vi "settings NM array.vi"(9 "Settings NM":dbl[](array[numeric]), 11 "Settings NM":T1 {"T8"."Medie" min=1 step=1; "T7"."Medie" min=1 step=1; "T6"."Medie" min=1 step=1; "T5"."Medie" min=1 step=1; "T4"."Medie" min=1 step=1; "T3"."Medie" min=1 step=1; "RM3"."Medie" min=1 step=1; "Tq3"."Medie" min=1 step=1; "Tq2"."Medie" min=1 step=1; "N3(T)"."Medie" min=1 step=1; "N2(T)"."Medie" min=1 step=1; "P10"."Medie" min=1 step=1; "P9"."Medie" min=1 step=1; "P8"."Medie" min=1 step=1; "P7"."Medie" min=1 step=1; "P6"."Medie" min=1 step=1; "P5"."Medie" min=1 step=1; "Q10"."Medie" min=1 step=1; "Q9"."Medie" min=1 step=1; "Q8"."Medie" min=1 step=1; "Q7"."Medie" min=1 step=1; "Q6"."Medie" min=1 step=1; "Q5"."Medie" min=1 step=1; "Pbar"."Medie" min=1 step=1; "Liv."."Medie" min=1 step=1; "RM2"."Medie" min=1 step=1; "RM1"."Medie" min=1 step=1; "T2"."Medie" min=1 step=1; "P4"."Medie" min=1 step=1; "Q4"."Medie" min=1 step=1; "RPM" items=["TESTO", "TORSIOMETRO", "OTTICA"]; "PRESSIONE\nMANDATA" items=["P1", "P2", "P3", "P4"]; "PRESSIONE\nASPIRAZIONE" items=["P1", "P2", "P3", "P4"]; "PORTATA\nSECONDARIA" items=["Q1", "Q2", "Q3", "Q4"]; "PORTATA\nPRINCIPALE" items=["LINEA ELETTROPOMPA", "LINEA SOMMERSA"]; "T1"."Medie" min=1 step=1; "Tq1"."Medie" min=1 step=1; "N1(T)"."Medie" min=1 step=1; "P3"."Medie" min=1 step=1; "P2"."Medie" min=1 step=1; "P1"."Medie" min=1 step=1; "Q3"."Medie" min=1 step=1; "Q2"."Medie" min=1 step=1; "Q1"."Medie" min=1 step=1}) -> (1 "Settings NM out":T1 {"T8"."Medie" min=1 step=1; "T7"."Medie" min=1 step=1; "T6"."Medie" min=1 step=1; "T5"."Medie" min=1 step=1; "T4"."Medie" min=1 step=1; "T3"."Medie" min=1 step=1; "RM3"."Medie" min=1 step=1; "Tq3"."Medie" min=1 step=1; "Tq2"."Medie" min=1 step=1; "N3(T)"."Medie" min=1 step=1; "N2(T)"."Medie" min=1 step=1; "P10"."Medie" min=1 step=1; "P9"."Medie" min=1 step=1; "P8"."Medie" min=1 step=1; "P7"."Medie" min=1 step=1; "P6"."Medie" min=1 step=1; "P5"."Medie" min=1 step=1; "Q10"."Medie" min=1 step=1; "Q9"."Medie" min=1 step=1; "Q8"."Medie" min=1 step=1; "Q7"."Medie" min=1 step=1; "Q6"."Medie" min=1 step=1; "Q5"."Medie" min=1 step=1; "Pbar"."Medie" min=1 step=1; "Liv."."Medie" min=1 step=1; "RM2"."Medie" min=1 step=1; "RM1"."Medie" min=1 step=1; "T2"."Medie" min=1 step=1; "P4"."Medie" min=1 step=1; "Q4"."Medie" min=1 step=1; "RPM" items=["TESTO", "TORSIOMETRO", "OTTICA"]; "PRESSIONE\nMANDATA" items=["P1", "P2", "P3", "P4"]; "PRESSIONE\nASPIRAZIONE" items=["P1", "P2", "P3", "P4"]; "PORTATA\nSECONDARIA" items=["Q1", "Q2", "Q3", "Q4"]; "PORTATA\nPRINCIPALE" items=["LINEA ELETTROPOMPA", "LINEA SOMMERSA"]; "T1"."Medie" min=1 step=1; "Tq1"."Medie" min=1 step=1; "N1(T)"."Medie" min=1 step=1; "P3"."Medie" min=1 step=1; "P2"."Medie" min=1 step=1; "P1"."Medie" min=1 step=1; "Q3"."Medie" min=1 step=1; "Q2"."Medie" min=1 step=1; "Q1"."Medie" min=1 step=1}, 3 "Settings NM out":dbl[](array[numeric]))   [LabVIEW 2019]
uses:
  TypeDef/cDAQ Settings NM.ctl
  TypeDef/SETUP INGRESSO.ctl
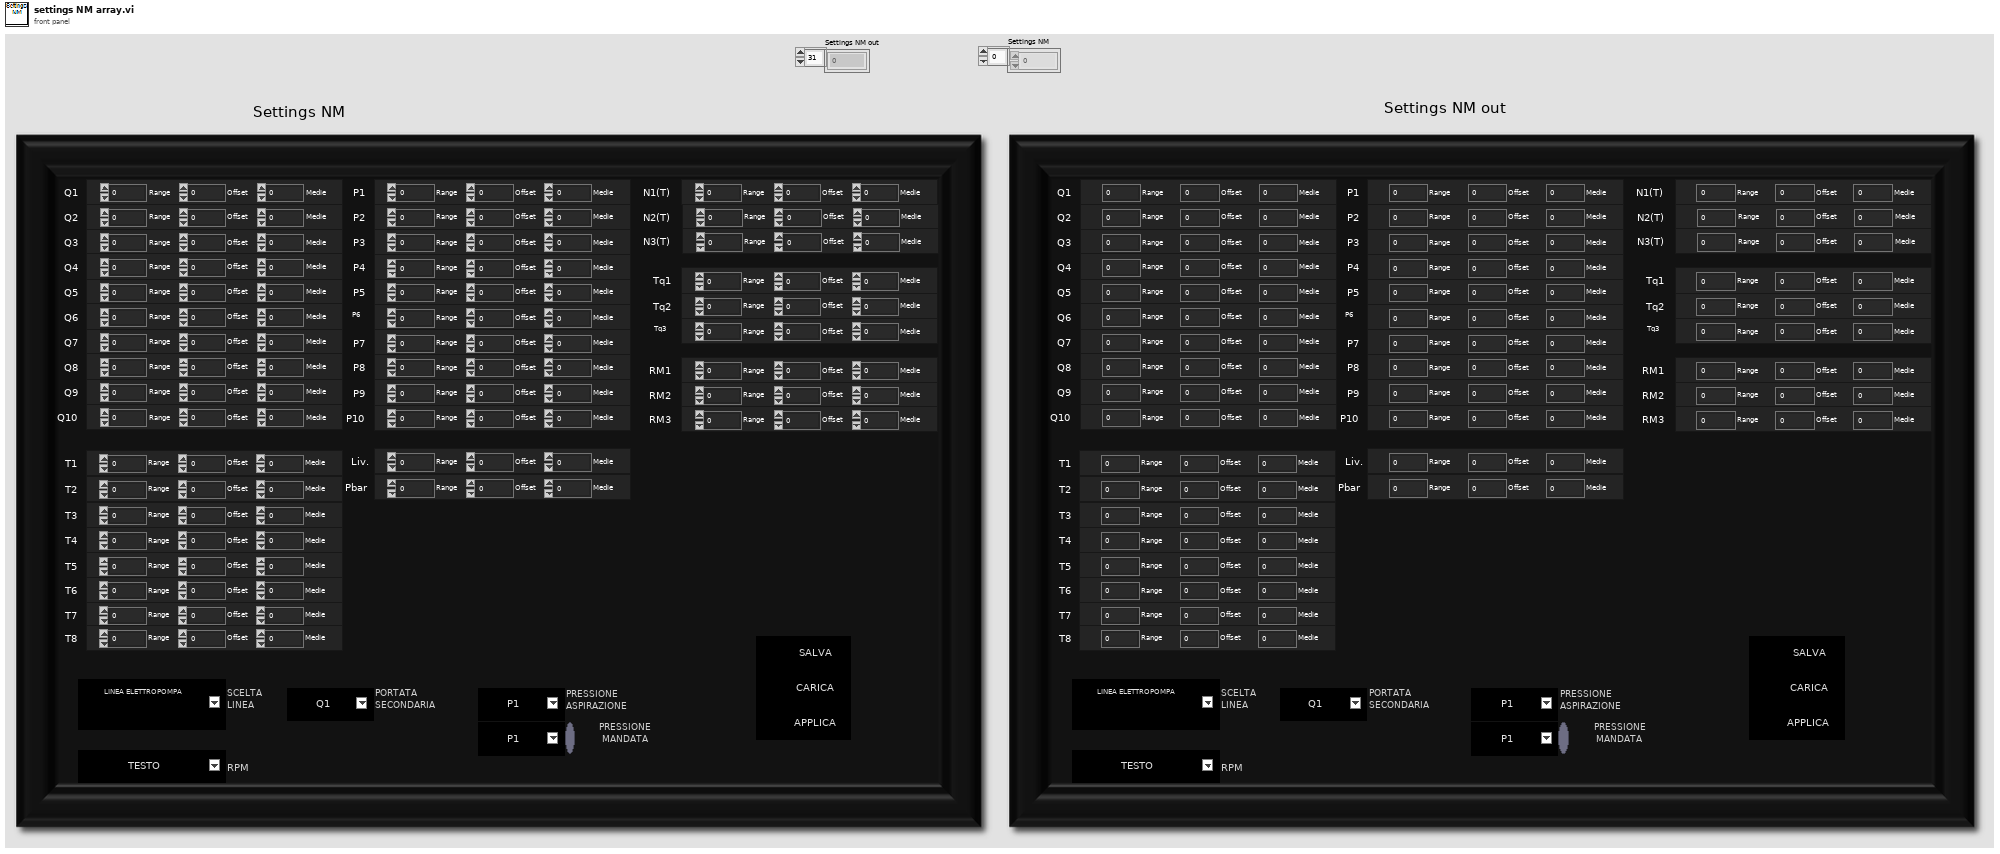
[diagram p1: front panel]
types:
  T1 = typedef "cDAQ Settings NM.ctl" = cluster{"SALVA":bool, "CARICA":bool, "APPLICA":bool, "Q1":T2, "Q2":T2, "Q3":T2, "Q4":T2, "Q5":T2, "Q6":T2, "Q7":T2, "Q8":T2, "Q9":T2, "Q10":T2, "P1":T2, "P2":T2, "P3":T2, "P4":T2, "P5":T2, "P6":T2, "P7":T2, "P8":T2, "P9":T2, "P10":T2, "N1(T)":T2, "N2(T)":T2, "N3(T)":T2, "Tq1":T2, "Tq2":T2, "Tq3":T2, "RM1":T2, "RM2":T2, "RM3":T2, "T1":T2, "T2":T2, "T3":T2, "T4":T2, "T5":T2, "T6":T2, "T7":T2, "T8":T2, "Liv.":T2, "Pbar":T2, "PORTATA\nPRINCIPALE":u16, "PORTATA\nSECONDARIA":u16, "PRESSIONE\nASPIRAZIONE":u16, "PRESSIONE\nMANDATA":u16, "RPM":u16, "differenziale?":bool}
  T2 = typedef "SETUP INGRESSO.ctl" = cluster{"Range":dbl, "Offset":dbl, "Medie":u8}
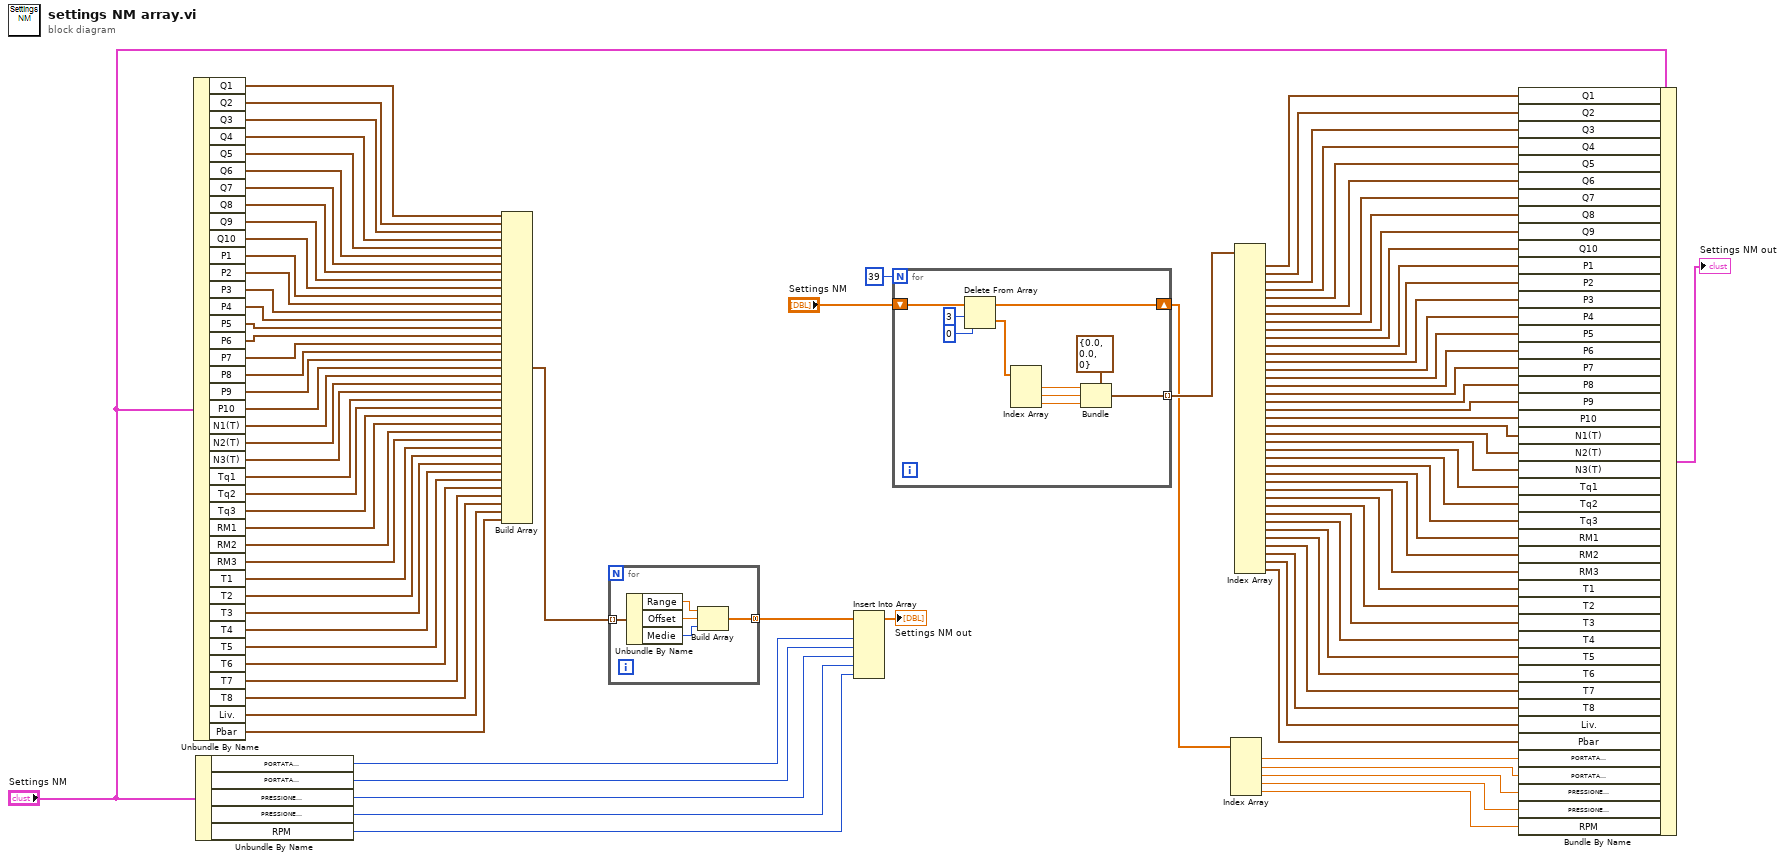
[diagram p0: block diagram]
diagram:
  n1 = Unbundle By Name("Settings NM") -> ("Q1"=w50:T2, "Q2"=w51:T2, "Q3"=w52:T2, "Q4"=w53:T2, "Q5"=w54:T2, "Q6"=w55:T2, "Q7"=w56:T2, "Q8"=w57:T2, "Q9"=w58:T2, "Q10"=w59:T2, "P1"=w60:T2, "P2"=w61:T2, "P3"=w62:T2, "P4"=w63:T2, "P5"=w64:T2, "P6"=w65:T2, "P7"=w66:T2, "P8"=w67:T2, "P9"=w68:T2, "P10"=w69:T2, "N1(T)"=w70:T2, "N2(T)"=w71:T2, "N3(T)"=w72:T2, "Tq1"=w73:T2, "Tq2"=w74:T2, "Tq3"=w75:T2, "RM1"=w76:T2, "RM2"=w77:T2, "RM3"=w78:T2, "T1"=w79:T2, "T2"=w80:T2, "T3"=w81:T2, "T4"=w82:T2, "T5"=w83:T2, "T6"=w84:T2, "T7"=w85:T2, "T8"=w86:T2, "Liv."=w87:T2, "Pbar"=w88:T2)
  n2 = Unbundle By Name("Settings NM") -> ("PORTATA\nPRINCIPALE"=w96:u16, "PORTATA\nSECONDARIA"=w95:u16, "PRESSIONE\nASPIRAZIONE"=w94:u16, "PRESSIONE\nMANDATA"=w93:u16, "RPM"=w92:u16)
  n3 = Build Array(w50, w51, w52, w53, w54, w55, w56, w57, w58, w59, w60, w61, w62, w63, w64, w65, w66, w67, w68, w69, w70, w71, w72, w73, w74, w75, w76, w77, w78, w79, w80, w81, w82, w83, w84, w85, w86, w87, w88) -> (w97:T2[])
  n4 = for {
    tunnel: w97 -> [w98] mode=indexing
    tunnel: [w99] -> w1 mode=concatenating
    n5 = Unbundle By Name(w98) -> ("Range"=w102:dbl, "Offset"=w101:dbl, "Medie"=w100:u8)
    n6 = Build Array(w102, w101, w100) -> (w99:dbl[])
  }
  n7 = Insert Into Array(array=w1, new element #1=w96, new element #2=w95, new element #3=w94, new element #4=w93, new element #5=w92) -> (→"Settings NM out":dbl[])  [unwired: 1 in]
  n8 = for {
    N: 39 -> [_]
    shift-right: [w109] -> w46
    shift-left: "Settings NM" -> [w112]
    tunnel: [w103] -> w47 mode=indexing
    n9 = Delete From Array(array=w112, length=3, index=0) -> (deleted portion=w107:dbl[], array with subset deleted=w109:dbl[])
    n10 = Index Array(array=w107) -> (element #1=w106:dbl, element #2=w105:dbl, element #3=w104:dbl)  [unwired: 3 in]
    n11 = Bundle(cluster=T2 {"Range"=0.0, "Offset"=0.0, "Medie"=0} ("Q1"), "Range"=w106, "Offset"=w105, "Medie"=w104) -> (w103:T2)
  }
  n12 = Index Array(array=w46) -> (element #1=w6:dbl, element #2=w5:dbl, element #3=w4:dbl, element #4=w3:dbl, element #5=w2:dbl)  [unwired: 5 in]
  n13 = Index Array(array=w47) -> (element #1=w45:T2, element #2=w44:T2, element #3=w43:T2, element #4=w42:T2, element #5=w41:T2, element #6=w40:T2, element #7=w39:T2, element #8=w38:T2, element #9=w37:T2, element #10=w36:T2, element #11=w35:T2, element #12=w34:T2, element #13=w33:T2, element #14=w32:T2, element #15=w31:T2, element #16=w30:T2, element #17=w29:T2, element #18=w28:T2, element #19=w27:T2, element #20=w26:T2, element #21=w25:T2, element #22=w24:T2, element #23=w23:T2, element #24=w22:T2, element #25=w21:T2, element #26=w20:T2, element #27=w19:T2, element #28=w18:T2, element #29=w17:T2, element #30=w16:T2, element #31=w15:T2, element #32=w14:T2, element #33=w13:T2, element #34=w12:T2, element #35=w11:T2, element #36=w10:T2, element #37=w9:T2, element #38=w8:T2, element #39=w7:T2)  [unwired: 39 in]
  n14 = Bundle By Name(cluster="Settings NM", "Q1"=w45, "Q2"=w44, "Q3"=w43, "Q4"=w42, "Q5"=w41, "Q6"=w40, "Q7"=w39, "Q8"=w38, "Q9"=w37, "Q10"=w36, "P1"=w35, "P2"=w34, "P3"=w33, "P4"=w32, "P5"=w31, "P6"=w30, "P7"=w29, "P8"=w28, "P9"=w27, "P10"=w26, "N1(T)"=w25, "N2(T)"=w24, "N3(T)"=w23, "Tq1"=w22, "Tq2"=w21, "Tq3"=w20, "RM1"=w19, "RM2"=w18, "RM3"=w17, "T1"=w16, "T2"=w15, "T3"=w14, "T4"=w13, "T5"=w12, "T6"=w11, "T7"=w10, "T8"=w9, "Liv."=w8, "Pbar"=w7, "PORTATA\nPRINCIPALE"=w6, "PORTATA\nSECONDARIA"=w5, "PRESSIONE\nASPIRAZIONE"=w4, "PRESSIONE\nMANDATA"=w3, "RPM"=w2) -> (→"Settings NM out":T1)
